vi "Unknown MSG Received from Target--error.vi"(10 "Data":string, 11 "Command":string) -> (0 "error out":errorcluster)   [LabVIEW 2021, in "Host Interpreter.lvlib"]
doc: "Outputs an error cluster containing a custom error code indicating the module is not running.\n_____\nBased on DQMH Dev Tools: Project Template 7.1.2.1547."
uses:
  Host Interpreter.lvlib
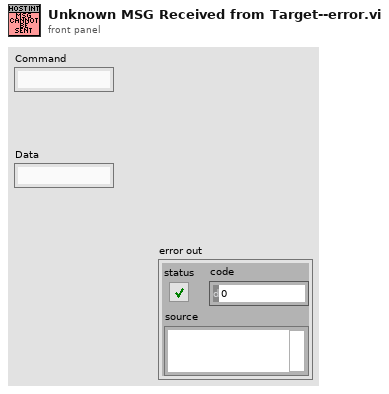
[diagram p1: front panel]
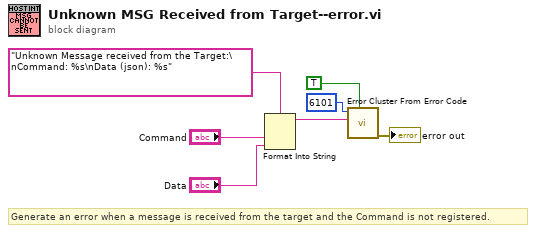
[diagram p0: block diagram]
diagram:
  # "Generate an error when a message is received from the target and the Command is not registered."
  n1 = Format Into String(format string="Unknown Message received from the Target:\nCommand: %s\nData (json): %s", "Command", "Data") -> (resulting string=w3:string)  [unwired: 2 in, 1 out]
  n2 = call <vilib>:"Error Cluster From Error Code.vi"("show call chain? (False)"=TRUE, "error message (\"\")"=w3, "error code (0)"=6101) -> ("error out"=→"error out":errorcluster)  [unwired: 6 in]
